vi "DMM Resistance Meas Format Measurement.vi"(0 "DMM Handle In":refnum<k15>, 5 "Measured Value":dbl, 7 "Function":i32, 9 "Digits Resolution":dbl, 11 "error in":errorcluster) -> (4 "DMM Handle Out":refnum<k15>, 6 "Measurement":string, 8 "Unit":string, 15 "error out":errorcluster)   [LabVIEW 2021, in "DMM_Resistance Measurement.lvlib"]
doc: "Converts the value measured by the niDMM Read into two output strings which contain the measurement and the correct units corresponding to the specific measurement."
uses:
  DMM_Resistance Measurement.lvlib
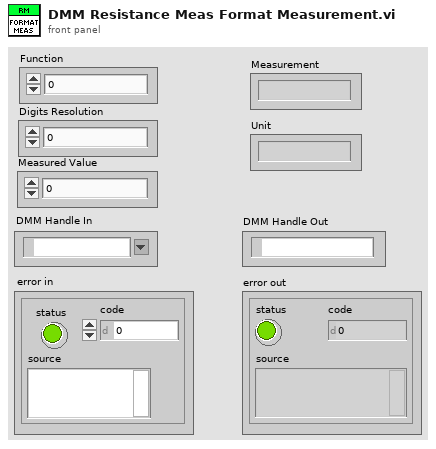
[diagram p1: front panel]
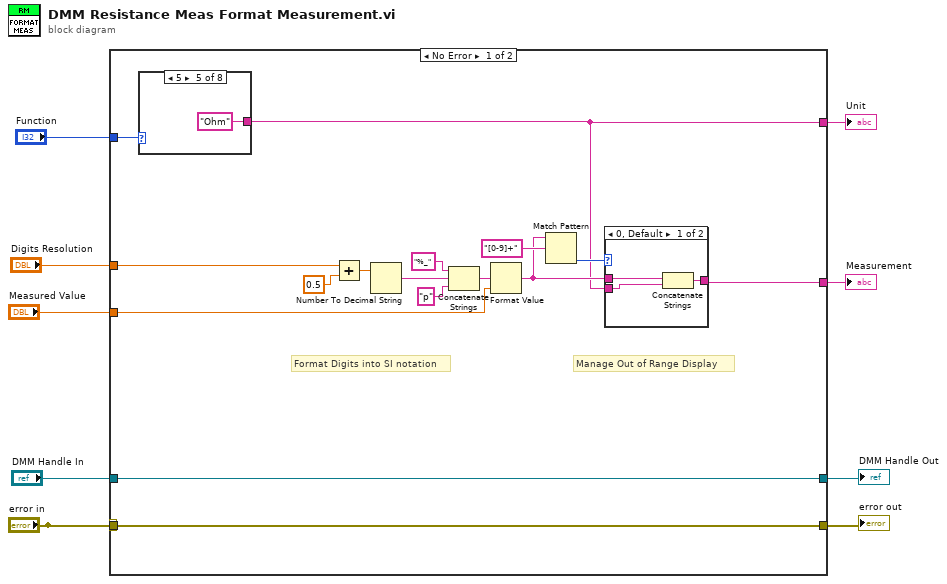
[diagram p0: block diagram]
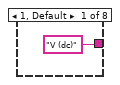
[diagram p3: hidden frame]
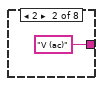
[diagram p4: hidden frame]
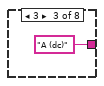
[diagram p5: hidden frame]
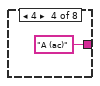
[diagram p6: hidden frame]
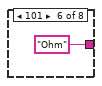
[diagram p7: hidden frame]
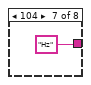
[diagram p8: hidden frame]
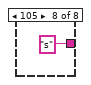
[diagram p9: hidden frame]
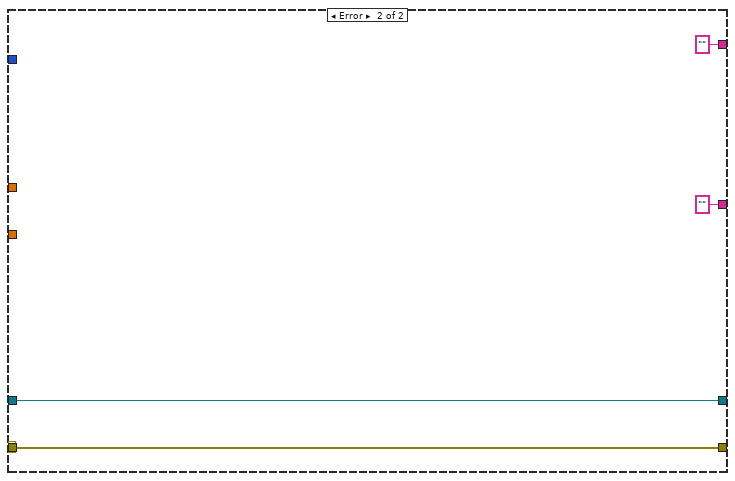
[diagram p10: hidden frame]
diagram:
  n1 = case shown="No Error" "error in" {
    tunnel: "error in" -> [w19 w41]
    tunnel: [w19 w41] -> w8
    tunnel: "DMM Handle In" -> [w18 w40]
    tunnel: [w18 w40] -> w6
    tunnel: "Function" -> [w17 _]
    tunnel: "Measured Value" -> [w16 _]
    tunnel: [w11 "" ("Units")] -> w3
    tunnel: [w10 ""] -> w2
    tunnel: "Digits Resolution" -> [w15 _]
    frame No Error {
      # "Manage Out of Range Display"
      # "Format Digits into SI notation"
      n2 = case shown="5" w17 {
        tunnel: ["V (dc)" ("Units") "V (ac)" ("Units") "A (dc)" ("Units") "A (ac)" ("Units") "Ohm" ("Units") "Ohm" ("Units") "Hz" ("Units") "s" ("Units")] -> w11
        frame 1, Default {
        }
        frame 2 {
        }
        frame 3 {
        }
        frame 4 {
        }
        frame 5 {
        }
        frame 101 {
        }
        frame 104 {
        }
        frame 105 {
        }
      }
      n3 = Add(x=w15, y=0.5) -> (x+y=w23:dbl)
      n4 = Number To Decimal String(number=w23) -> (decimal integer string=w24:string)  [unwired: 1 in]
      n5 = Concatenate Strings("%_" ("string"), w24, "p" ("string")) -> (w25:string)
      n6 = Format Value(format string=w25, value (0)=w16) -> (output string=w12:string)  [unwired: 1 in]
      n7 = Match Pattern(string=w12, regular expression="[0-9]+") -> (offset past match=w13:i32)  [unwired: 1 in, 3 out]
      n8 = case shown="0, Default" w13 {
        tunnel: w12 -> [w26 w29]
        tunnel: w11 -> [w28 _]
        tunnel: [w27 w29] -> w10
        frame 0, Default {
          n9 = Concatenate Strings(w26, w28) -> (w27:string)
        }
        frame -1 {
        }
      }
    }
    frame Error {
    }
  }
  "error out" <- w8
  "DMM Handle Out" <- w6
  "Unit" <- w3
  "Measurement" <- w2
